vi "Prober_ThetaAlignment.vi"(4 "y2":dbl, 5 "y1":dbl, 6 "x2":dbl, 7 "x1":dbl, 8 "error in (no error)":errorcluster, 11 "ProbeStationControl in":refnum<class "ProbeStationControl.lvclass">) -> (0 "error out":errorcluster, 1 "theta increment":i32, 2 "New millidegrees":i32, 3 "ProbeStationControl out":refnum<class "ProbeStationControl.lvclass">)   [LabVIEW 2018, in "ProbeStationControl.lvclass"]
uses:
  ProbeStationControl.lvclass
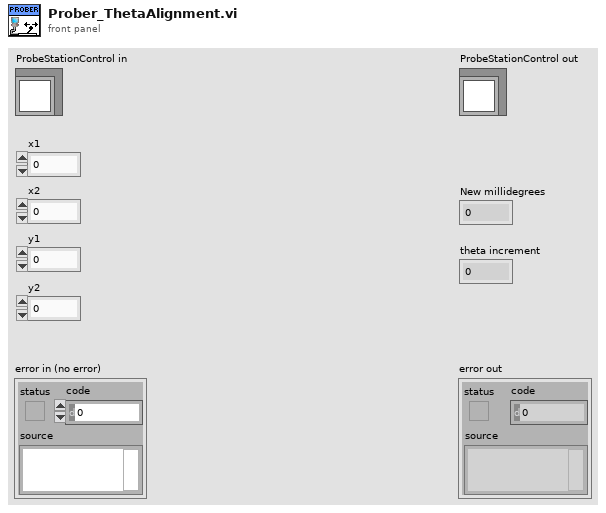
[diagram p1: front panel]
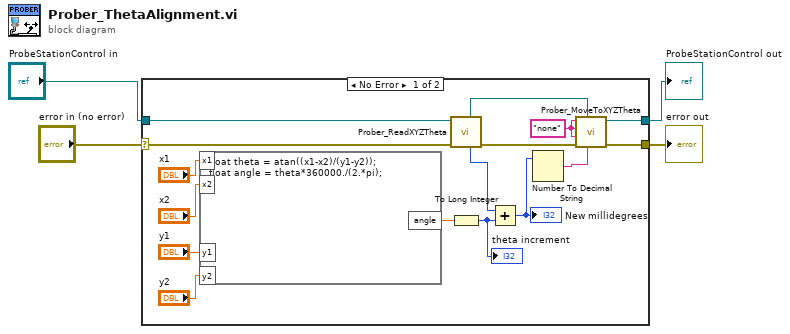
[diagram p0: block diagram]
diagram:
  n1 = case shown="No Error" "error in (no error)" {
    selector: "error in (no error)" -> [w15 w22]
    tunnel: [w7 w22] -> w3
    tunnel: [w8 w21] -> w1
    tunnel: "ProbeStationControl in" -> [w16 w21]
    frame No Error {
      w12 = "none"
      n2 = formula code="float theta = atan((x1-x2)/(y1-y2));\nfloat angle = theta*360000./(2.*pi);"("x1"="x1", "x2"="x2", "y1"="y1", "y2"="y2") -> ("angle"=w13:dbl)
      n3 = call "Prober_ReadXYZTheta.vi"("error in (no error)"=w15, "ProbeStationControl in"=w16) -> ("error out"=w9:errorcluster, "Theta location [mdeg]"=w14:i32, "ProbeStationControl out"=w10:refnum<class "ProbeStationControl.lvclass">)  [unwired: 4 in, 3 out]
      n4 = To Long Integer(number=w13) -> (32bit integer=w5:i32)
      "theta increment" <- w5
      n5 = Add(x=w14, y=w5) -> (x+y=w6:i32)
      "New millidegrees" <- w6
      n6 = Number To Decimal String(number=w6) -> (decimal integer string=w11:string)  [unwired: 1 in]
      n7 = call "Prober_MoveToXYZTheta.vi"("Theta location [mdeg]"=w11, "ProbeStationControl in"=w10, "error in (no error)"=w9, "Z location [µm]"=w12, "Y location [µm]"=w12, "X location [µm]"=w12) -> ("error out"=w7:errorcluster, "ProbeStationControl out"=w8:refnum<class "ProbeStationControl.lvclass">)  [unwired: 3 in, 1 out]
    }
    frame Error {
    }
  }
  "error out" <- w3
  "ProbeStationControl out" <- w1
